vi "Module ID.vi"(11 "Telemetry Command Module in":refnum<class "Telemetry Command Module.lvclass">) -> (2 "Module ID":string)   [LabVIEW 2020, in "VolatusGUI.lvlib" / "Telemetry Command Module.lvclass"]
uses:
  Telemetry Command Module.lvclass
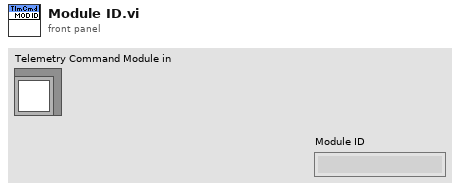
[diagram p1: front panel]
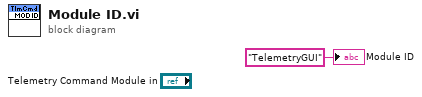
[diagram p0: block diagram]
diagram:
  "Module ID" <- "TelemetryGUI" ("Module ID")
